vi "Trigger Detection for 1 Channel.vi"(0 "signal in":waveform(dbl), 1 "reset":bool, 5 "level":dbl format="%.2p", 7 "hysteresis":dbl format="%.2p", 9 "location mode":u16(ring) items=["Index", "Time"], 11 "error in (no error)":errorcluster, 12 "trigger slope":u16(ring)=1 items=["Falling Edge", "Rising Edge"]) -> (4 "trigger location":dbl format="%#_2g", 6 "trigger detected?":bool, 15 "error out":errorcluster)   [LabVIEW 2020, in "NI_MAPro.lvlib"]
doc: "Finds the first level-crossing location in a waveform. You can retrieve the trigger location as an index or as a time. The trigger conditions are specified in terms of threshold <B>level</B>, <B>slope</B>, and <B>hysteresis</B>. Wire data to the <B>signal in</B> input to determine the polymorphic instance to use or manually select the instance."
uses:
  NI_MAPro.lvlib
  NI_MABase.lvlib
  <resource>/lvanlys.dll
panel:
  out "number of triggers detected":i32
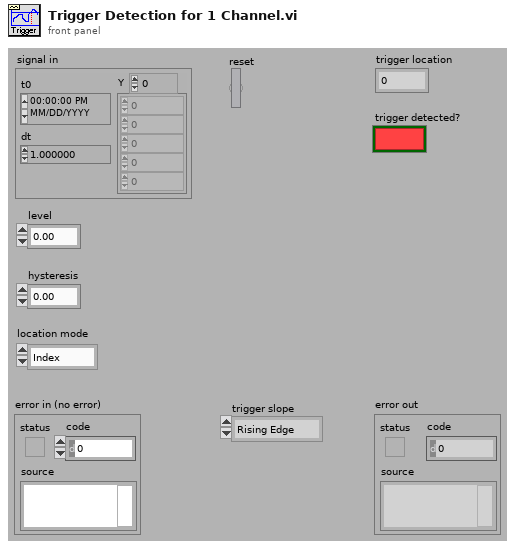
[diagram p1: front panel]
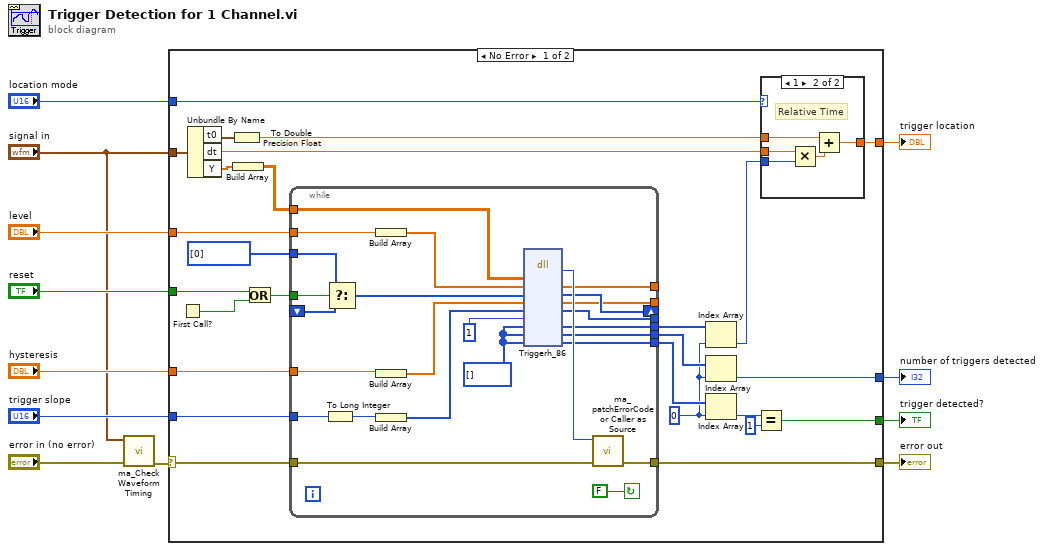
[diagram p0: block diagram]
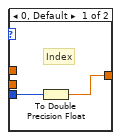
[diagram p2: hidden frame]
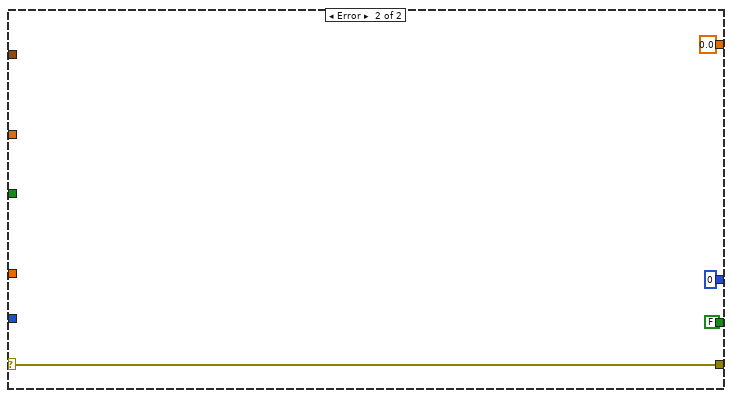
[diagram p3: hidden frame]
diagram:
  n1 = call "ma_Check Waveform Timing.vi"("error in (no error)"="error in (no error)", "signal in"="signal in") -> ("error out"=w10:errorcluster)  [unwired: 1 in, 8 out]
  n2 = case shown="No Error" w10 {
    selector: w10 -> [w38 w74]
    tunnel: [w37 w74] -> w12
    tunnel: "signal in" -> [w18 _]
    tunnel: "hysteresis" -> [w36 _]
    tunnel: "trigger slope" -> [w35 _]
    tunnel: "reset" -> [w34 _]
    tunnel: "level" -> [w30 _]
    tunnel: [w29 0.0] -> w3
    tunnel: [w22 0] -> w2
    tunnel: [w21 FALSE] -> w5
    tunnel: "location mode" -> [w19 _]
    frame No Error {
      w24 = 0 ("Index")
      n3 = First Call?() -> (First Call?: T/F=w33:bool)
      n4 = Unbundle By Name(w18) -> ("t0"=w17:timestamp, "dt"=w15:dbl, "Y"=w14:dbl[])
      n5 = To Double Precision Float(number=w17) -> (double precision float=w16:dbl)
      n6 = Build Array(w14) -> (w13:dbl[][])
      n7 = Or(x=w34, y=w33) -> (x .or. y?=w32:bool)
      n8 = while {
        tunnel: w38 -> [w63]
        tunnel: [w62] -> w37
        shift-right: [w69] -> _
        shift-left: _ -> [w59]
        tunnel: w36 -> [w57]
        tunnel: w35 -> [w56]
        tunnel: w32 -> [w55]
        tunnel: i32[] [0] -> [w54]
        tunnel: w30 -> [w53]
        tunnel: [w52] -> w27
        tunnel: [w51] -> w26
        tunnel: [w50] -> w25
        tunnel: w13 -> [w49]
        tunnel: [w48] -> _
        tunnel: [w47] -> _
        tunnel: [w46] -> _
        stop <- FALSE continue-if-true
        w58 = i32[] [] ("Array Constant")
        n9 = To Long Integer(number=w56) -> (32bit integer=w65:i32)
        n10 = Select(t=w54, s=w55, f=w59) -> (s? t:f=w60:i32[])
        n11 = Build Array(w53) -> (w67:dbl[])
        n12 = Build Array(w57) -> (w66:dbl[])
        n13 = Build Array(w65) -> (w61:i32[])
        n14 = dll-call lib="C:/Program Files (x86)/National Instruments/LabVIEW 2020/resource/lvanlys.*" fn="Triggerh_86"("x"=w49, "level"=w67, "status"=w60, "hysterisis"=w66, "slope"=w61, "nptsH"=1 ("max number trigger pts"), "triggerIndex"=w58, "number_of_triggers_detected"=w58, "triggerDetectedbyte"=w58) -> ("return type"=w70:i32, "level"=w48:dbl[], "status"=w69:i32[], "hysterisis"=w47:dbl[], "slope"=w46:i32[], "triggerIndex"=w52:i32[], "number_of_triggers_detected"=w51:i32[], "triggerDetectedbyte"=w50:i32[])  [unwired: 5 in, 2 out]
        n15 = call "ma_patchErrorCode or Caller as Source.vi"("error in (no error)"=w63, "error code"=w70) -> ("error out"=w62:errorcluster)  [unwired: 2 in, 7 out]
      }
      n16 = Index Array(array=w27, index=w24) -> (element=w20:i32)
      n17 = Index Array(array=w26, index=w24) -> (element=w22:i32)
      n18 = Index Array(array=w25, index=w24) -> (element=w28:i32)
      n19 = Equal?(x=w28, y=1 ("Element Data")) -> (x = y?=w21:bool)
      n20 = case shown="1" w19 {
        tunnel: w20 -> [w40 w45]
        tunnel: [w39 w41] -> w29
        tunnel: w15 -> [_ w44]
        tunnel: w16 -> [_ w42]
        frame 0, Default {
          # "Index"
          n21 = To Double Precision Float(number=w40) -> (double precision float=w39:dbl)
        }
        frame 1 {
          # "Relative Time"
          n22 = Multiply(x=w44, y=w45) -> (x*y=w43:dbl)
          n23 = Add(x=w42, y=w43) -> (x+y=w41:dbl)
        }
      }
    }
    frame Error {
    }
  }
  "error out" <- w12
  "trigger detected?" <- w5
  "trigger location" <- w3
  "number of triggers detected" <- w2
